vi "Blink.vi"() -> ()   [LabVIEW 2018]
panel:
  out "Boolean 2":bool
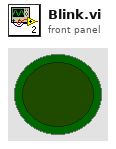
[diagram p1: front panel]
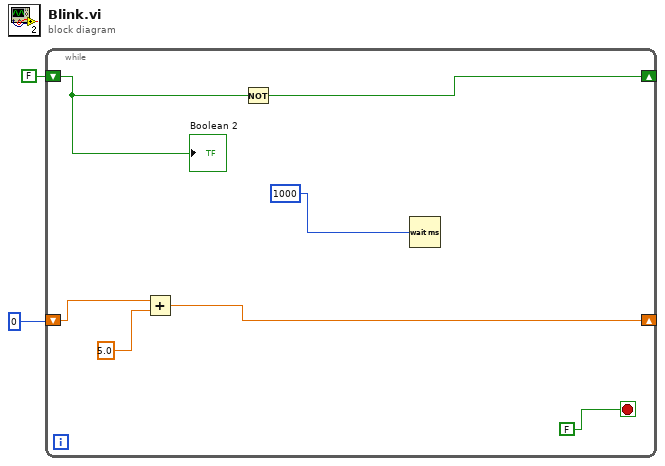
[diagram p0: block diagram]
diagram:
  n1 = while {
    shift-right: [w9] -> _
    shift-left: FALSE -> [w8]
    shift-right: [w4] -> _
    shift-left: 0 -> [w5]
    stop <- FALSE stop-if-true
    n2 = Add(x=w5, y=5.0) -> (x+y=w4:dbl)
    n3 = Not(x=w8) -> (.not. x?=w9:bool)
    n4 = Wait (ms)(milliseconds to wait=1000) -> ()  [unwired: 1 out]
    "Boolean 2" <- w8
  }
